vi "TCP_通讯状态.vi"(7 "写入地址":u32=1000, 9 "写入数据":i8) -> (3 "状态":bool)   [LabVIEW 2013]
uses:
  S7Ref.vi
panel:
  in  "error in (no error)":errorcluster
  out "error out":errorcluster
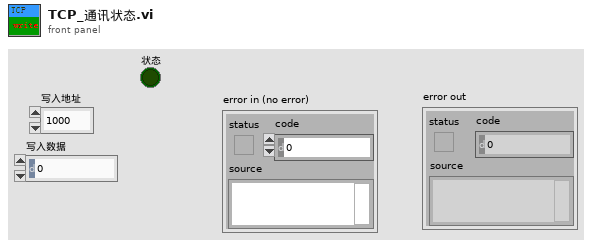
[diagram p1: front panel]
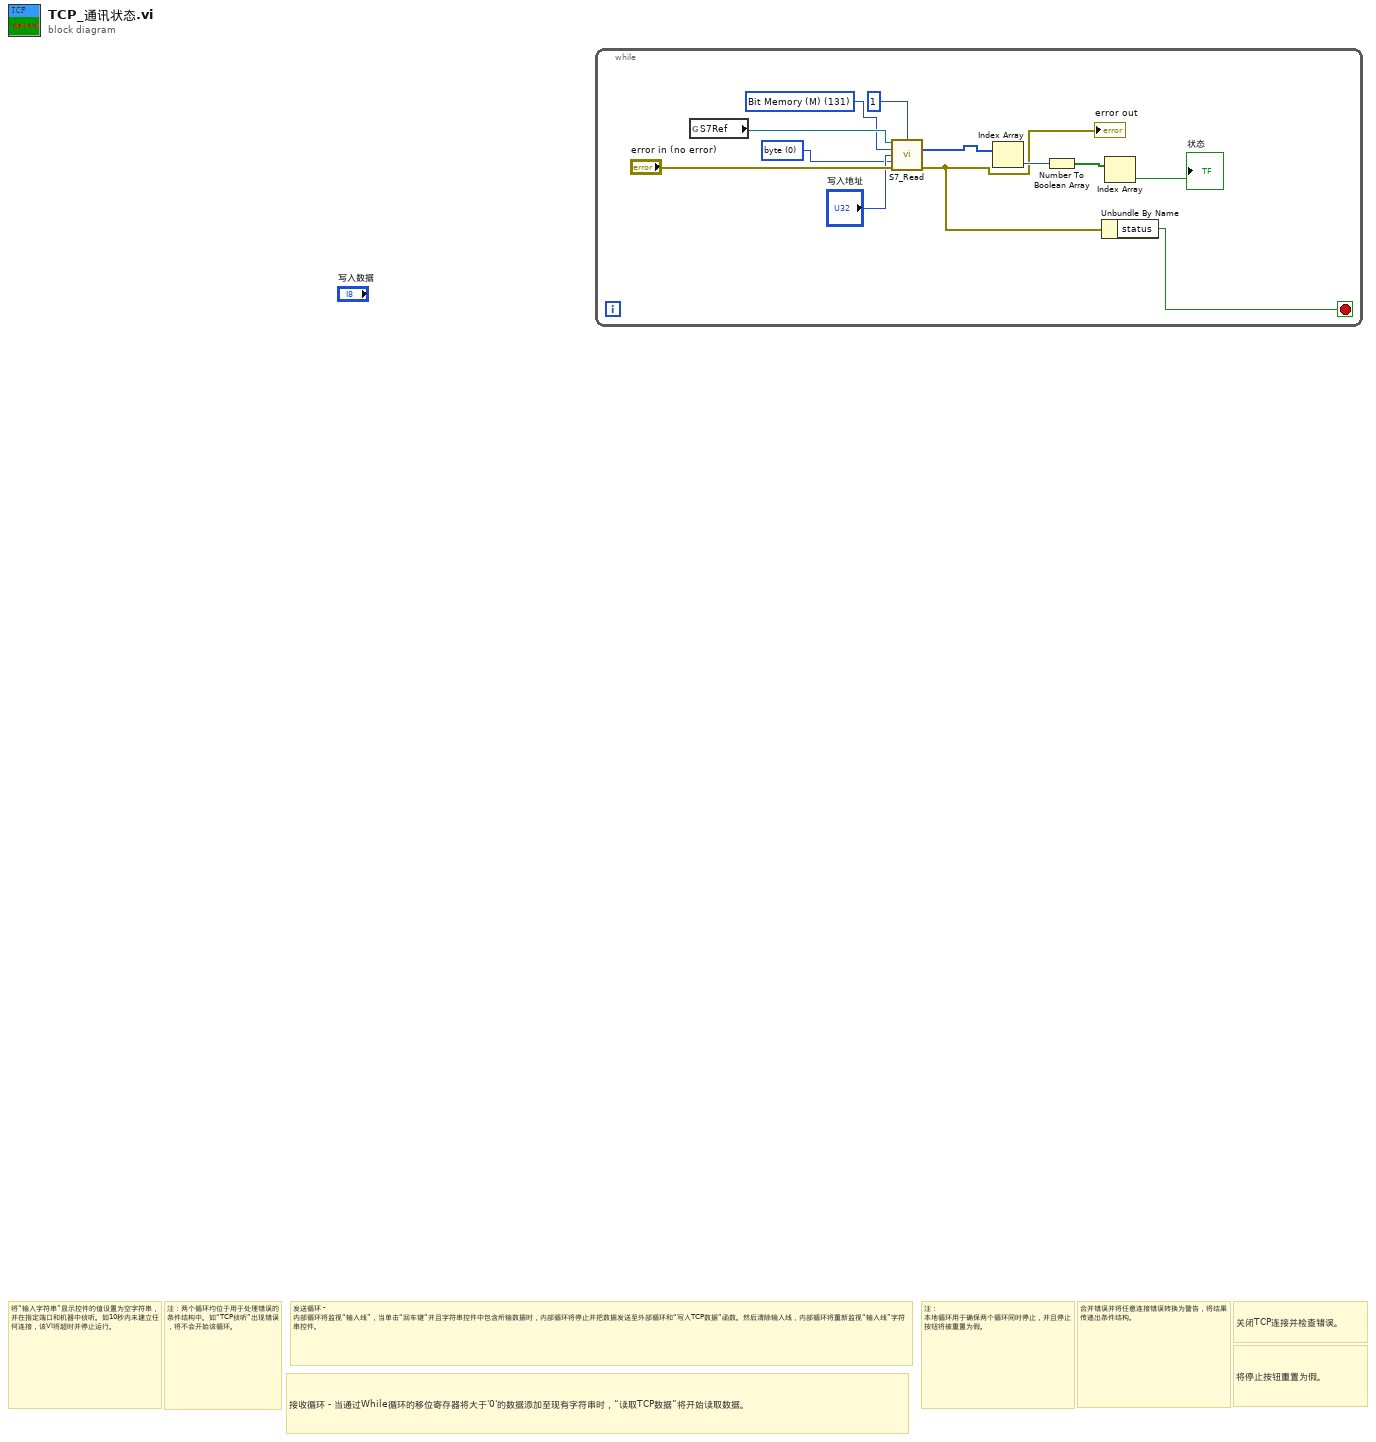
[diagram p0: block diagram]
diagram:
  # "将停止按钮重置为假。"
  # "关闭TCP连接并检查错误。"
  # "注：两个循环均位于用于处理错误的条件结构中。如“TCP侦听”出现错误，将不会开始该循环。"
  # "合并错误并将任意连接错误转换为警告，将结果传递出条件结构。"
  # "注： 本地循环用于确保两个循环同时停止，并且停止按钮将被重置为假。"
  # "接收循环 - 当通过While循环的移位寄存器将大于'0'的数据添加至现有字符串时，“读取TCP数据”将开始读取数据。"
  # "发送循环 - 内部循环将监视“输入线”，当单击“回车键”并且字符串控件中包含所输数据时，内部循环将停止并把数据发送至外部循环和“写入TCP数据”函数。然后清除输入线，内部循环将重新监视“输入线”字符串控件。"
  # "将“输入字符串”显示控件的值设置为空字符串，并在指定端口和机器中侦听。如10秒内未建立任何连接，该VI将超时并停止运行。"
  n1 = while {
    stop <- w1 stop-if-true
    w8 = u16 0 items=["byte", "word", "Dword"] ("数据类型")
    w6 = u8 131 items=["I/O (P)"=128, "Input (I)"=129, "Output (Q)"=130, "Bit Memory (M)"=131, "Data (DB)"=132, "Instance Data (DI)"=133, "Local Data (L)"=134, "Predecessor Local Data (VL)"=135] ("寄存器类型")
    n2 = global read "S7Ref.vi" "S7Ref"() -> (w11:refnum<k5>)
    n3 = call "S7_Read .vi"("TCP"=w11, "读取长度"=u16 1, "寄存器类型"=w6, "起始地址"="写入地址", "数据类型"=w8, "error in"="error in (no error)") -> ("数据"=w5:u32[], "error out"=w2:errorcluster)  [unwired: 6 in, 2 out]
    "error out" <- w2
    n4 = Index Array(array=w5) -> (element=w9:u32)  [unwired: 1 in]
    n5 = Number To Boolean Array(number=w9) -> (Boolean array=w4:bool[])
    n6 = Unbundle By Name(w2) -> ("status"=w1:bool)
    n7 = Index Array(array=w4) -> (element=→"状态":bool)  [unwired: 1 in]
  }
